vi "1_acq_To_ArrayU8.vi"(0 "File path":path, 2 "Frame":u32, 5 "error in":errorcluster) -> (14 "Array Src OUT":u8[](array[numeric]), 15 "Array Dst OUT":u8[](array[numeric]), 17 "Width":i32, 18 "Height":i32, 19 "Error Out":errorcluster)   [LabVIEW 2018]
doc: "It reads an .acq file and it returns the 1D array U8 of the source image, the 1D array U8 that will save the destination image, the width and height of the image. It It receives the path of an .acq file and the desired internal frame number."
uses:
  Controls/DataLog_Data_Type.ctl
panel:
  in  "DataLog_Data_Type 2":T1
  in  "DataLog_Data_Type":T1
  out "IMG":u8[][](array[numeric])
  out "Number of IMGs":u32
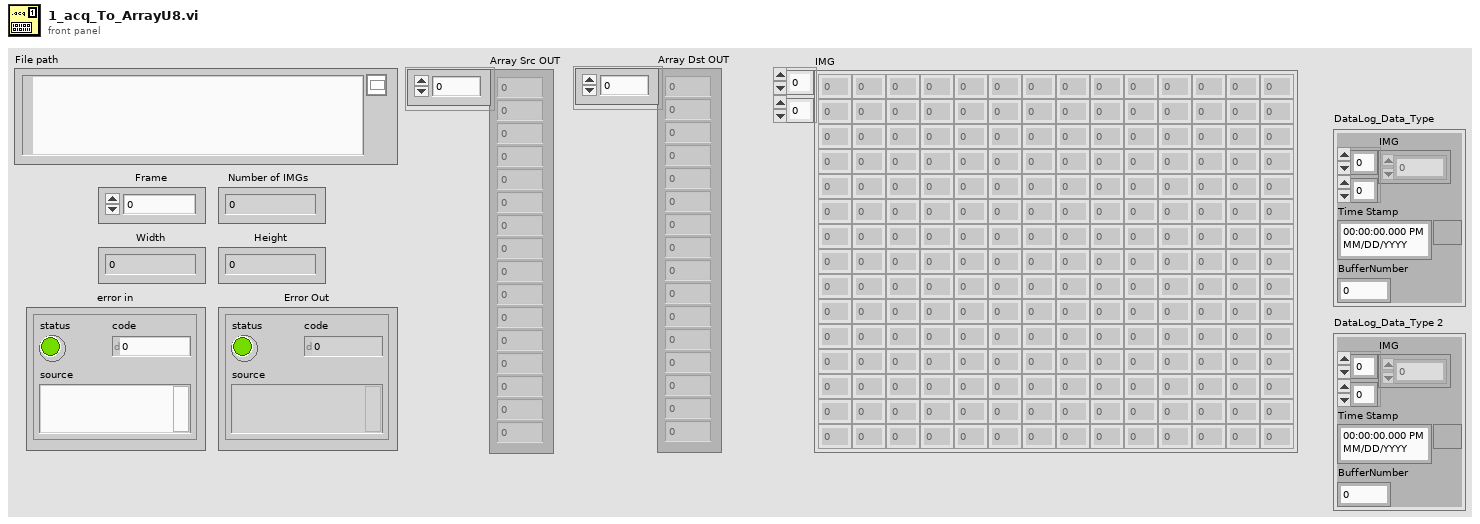
[diagram p1: front panel]
types:
  T1 = typedef "DataLog_Data_Type.ctl" = cluster{"IMG":u8[][], "Time Stamp":timestamp, "BufferNumber":u32}
  T2 = enum16{"open", "replace", "create", "open or create", "replace or create", "replace or create with confirmation"}
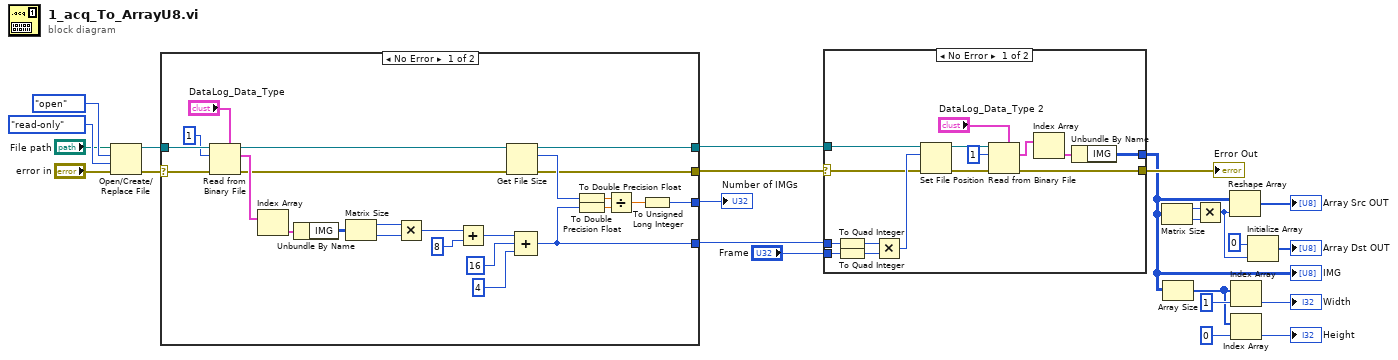
[diagram p0: block diagram]
diagram:
  n1 = Open/Create/Replace File(file path (use dialog)="File path", error in="error in", operation (0:open)=T2."open", access (0:read/write)=enum16{"read/write", "read-only", "write-only"}."read-only") -> (refnum out=w9:refnum<file>, error out=w8:errorcluster)  [unwired: 2 in, 1 out]
  n2 = case shown="No Error" w8 {
    selector: w8 -> [w42 w49]
    tunnel: [w36 w49] -> w5
    tunnel: w9 -> [w45 w50]
    tunnel: [w44 w50] -> w6
    tunnel: [w35 _] -> w7
    tunnel: [w25 _] -> w3
    frame No Error {
      n3 = Read from Binary File(5:"DataLog_Data_Type", 8:w42, 10:1 ("count (1)"), 11:w45) -> (0:w34:errorcluster, 2:w40:T1[], 3:w43:refnum<file>)  [unwired: 2 in, 1 out]
      n4 = Index Array(array=w40) -> (element=w39:T1)  [unwired: 1 in]
      n5 = Unbundle By Name(w39) -> ("IMG"=w38:u8[][])
      n6 = Matrix Size(0:w38) -> (1:w27:i32, 2:w26:i32)
      n7 = Multiply(x=w27, y=w26) -> (x*y=w29:i32)
      n8 = Add(x=w29, y=8) -> (x+y=w31:i32)
      n9 = Get File Size(file=w43, error in=w34) -> (refnum out=w44:refnum<file>, size (in bytes)=w46:i64, 0:w36:errorcluster)
      n10 = Compound Arithmetic op=ADD(w31, 16 ("y"), 4 ("y")) -> (w25:i32)
      n11 = To Double Precision Float(number=w46) -> (double precision float=w47:dbl)
      n12 = To Double Precision Float(number=w25) -> (double precision float=w48:dbl)
      n13 = Divide(x=w47, y=w48) -> (x/y=w37:dbl)
      n14 = To Unsigned Long Integer(number=w37) -> (unsigned 32bit integer=w35:u32)
    }
    frame Error {
    }
  }
  "Number of IMGs" <- w7
  n15 = case shown="No Error" w5 {
    selector: w5 -> [w52 w66]
    tunnel: [w63 _] -> w1
    tunnel: "Frame" -> [w59 _]
    tunnel: w3 -> [w57 _]
    tunnel: [w56 w66] -> w2
    tunnel: w6 -> [w53 _]
    frame No Error {
      n16 = To Quad Integer(1:w57) -> (0:w64:i64)
      n17 = To Quad Integer(1:w59) -> (0:w65:i64)
      n18 = Multiply(x=w64, y=w65) -> (x*y=w58:i64)
      n19 = Set File Position(offset (in bytes) (0)=w58, refnum=w53, error in=w52) -> (refnum out=w54:refnum<file>, error out=w55:errorcluster)  [unwired: 1 in]
      n20 = Read from Binary File(5:"DataLog_Data_Type 2", 8:w55, 10:1 ("count (1)"), 11:w54) -> (0:w56:errorcluster, 2:w60:T1[])  [unwired: 2 in, 2 out]
      n21 = Index Array "Index Array"(array=w60) -> (element=w62:T1)  [unwired: 1 in]
      n22 = Unbundle By Name(w62) -> ("IMG"=w63:u8[][])
    }
    frame Error {
    }
  }
  "Error Out" <- w2
  "IMG" <- w1
  n23 = Matrix Size(0:w1) -> (1:w19:i32, 2:w20:i32)
  n24 = Array Size(array=w1) -> (size(s)=w12:i32[])
  n25 = Multiply(x=w19, y=w20) -> (x*y=w16:i32)
  n26 = Reshape Array(w1, w16) -> (→"Array Src OUT":u8[])
  n27 = Index Array(array=w12, index=1) -> (element=→"Width":i32)
  n28 = Index Array(array=w12, index=0) -> (element=→"Height":i32)
  n29 = Initialize Array(u8 0 ("element"), w16) -> (→"Array Dst OUT":u8[])
